vi "DHE_DRV_manual_command.vi"(0 "arg3":string, 1 "arg4":string, 2 "arg5":string, 3 "command":string, 4 "short board_dest":i16, 5 "error in (no error)":errorcluster, 6 "arg2":string, 8 "arg1":string, 10 "fd":i32) -> (14 "fd":i32, 18 "error_code":i32, 19 "error out":errorcluster)   [LabVIEW 2016]
doc: "This VI closes the I/O interface with the instrument."
uses:
  c/lib/libarcDHE.so
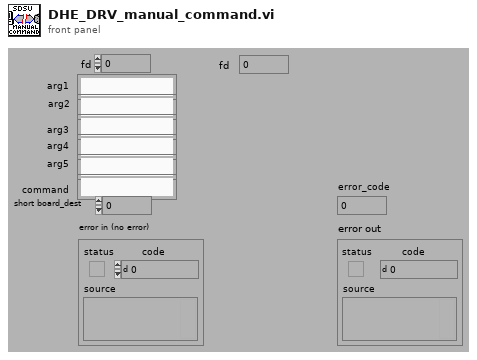
[diagram p1: front panel]
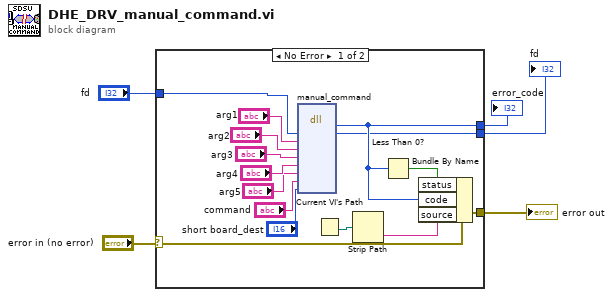
[diagram p0: block diagram]
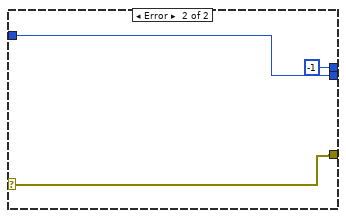
[diagram p2: hidden frame]
diagram:
  n1 = case shown="No Error" "error in (no error)" {
    selector: "error in (no error)" -> [w7 w23]
    tunnel: [w19 -1] -> w5
    tunnel: [w16 w23] -> w4
    tunnel: [w15 w22] -> w3
    tunnel: "fd" -> [w6 w22]
    frame No Error {
      n2 = dll-call lib="home/simager/panview/PAN/Modules/SDSU/private/c/lib/libarcDHE.so" fn="manual_command" label="manual command"("fd"=w6, "arg1"="arg1", "arg2"="arg2", "arg3"="arg3", "arg4"="arg4", "arg5"="arg5", "command"="command", "short board_dest"="short board_dest") -> (w19:i32, "fd"=w15:i32)  [unwired: 10 in, 2 out]
      n3 = Current VI's Path() -> (path=w18:path)
      n4 = Strip Path(path=w18) -> (name=w17:string)  [unwired: 1 out]
      n5 = Less Than 0?(x=w19) -> (x < 0?=w20:bool)
      n6 = Bundle By Name(cluster=w7, "status"=w20, "code"=w19, "source"=w17) -> (w16:errorcluster)
    }
    frame Error {
    }
  }
  "error out" <- w4
  "error_code" <- w5
  "fd" <- w3
